vi "SetupTimerPanel.vi"(0 "VI in":refnum<vi>, 5 "Item Name":string, 11 "error in (no error)":errorcluster, 12 "milliseconds to wait (1000)":u32=1000) -> (4 "VI out":refnum<vi>, 15 "error out":errorcluster)   [LabVIEW 2016, in "DronaTest.lvlib"]
uses:
  DronaTest.lvlib
  APIs/Assert/AssertSubpanel/AssertSubpanelVIExecRunning.vi
  APIs/Stimulus/ControlValue/ValueSignalLatchBooleanString.vi
  Drona.lvlib
  APIs/Assert/AssertSubpanel/AssertSubpanel.lvlib
  APIs/Stimulus/ControlValue/ControlValue.lvlib
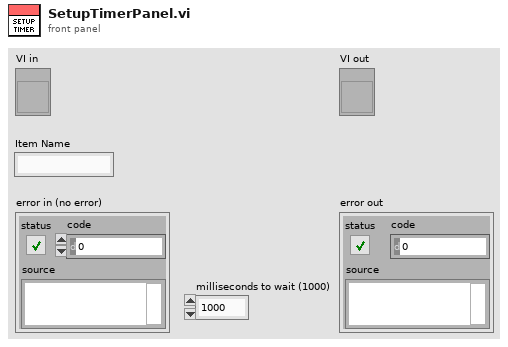
[diagram p1: front panel]
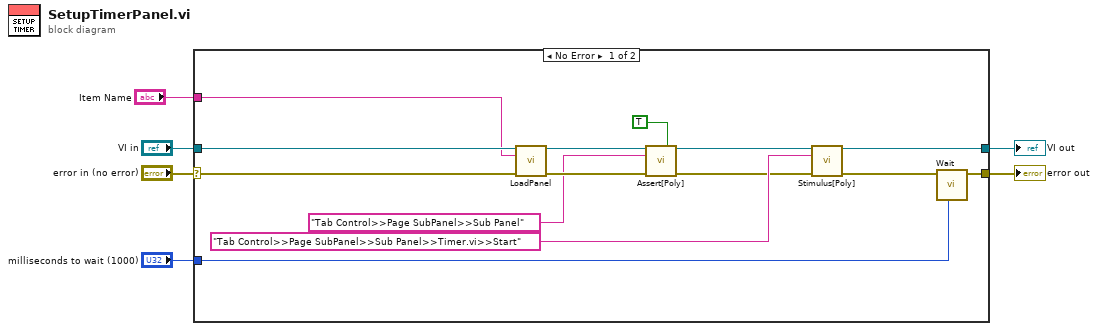
[diagram p0: block diagram]
diagram:
  n1 = case shown="No Error" "error in (no error)" {
    selector: "error in (no error)" -> [w20 w21]
    tunnel: "VI in" -> [w19 w22]
    tunnel: [w12 w22] -> w4
    tunnel: [w9 w21] -> w3
    tunnel: "milliseconds to wait (1000)" -> [w8 _]
    tunnel: "Item Name" -> [w7 _]
    frame No Error {
      n2 = call "LoadPanel.vi"("VI in"=w19, "Item Name"=w7, "error in"=w20) -> ("VI out"=w17:refnum<vi>, "error out"=w18:errorcluster)  [unwired: 11 in]
      n3 = call-poly "Assert[Poly].vi"("VI Reference In"=w17, "Assert Only? (F)"=TRUE, "Control Path"="Tab Control>>Page SubPanel>>Sub Panel", "Error In"=w18) -> ("VI Reference Out"=w13:refnum<vi>, "Error Out"=w11:errorcluster)  [unwired: 9 in, 1 out]
      n4 = call-poly "Stimulus[Poly].vi"("VI Reference In"=w13, "Control Path"="Tab Control>>Page SubPanel>>Sub Panel>>Timer.vi>>Start", "error in"=w11) -> ("VI Reference Out"=w12:refnum<vi>, "error out"=w10:errorcluster)  [unwired: 11 in]
      n5 = call "Wait.vi"("milliseconds to wait"=w8, "error in (no error)"=w10) -> ("error out"=w9:errorcluster)  [unwired: 9 in]
    }
    frame Error {
    }
  }
  "error out" <- w3
  "VI out" <- w4
